vi "Measurement Logic.vi"() -> ()   [LabVIEW 2021, in "Line Regulation_Channel Ganging.lvlib"]
uses:
  Line Regulation_Channel Ganging.lvlib
  Measurement Results.ctl
  <instrlib>/niDCPower/nidcpower.llb/niDCPower Source Mode.ctl
  <instrlib>/niDCPower/nidcpower.llb/niDCPower Output Function.ctl
  <instrlib>/niDCPower/nidcpower.llb/niDCPower Wait For Event - Event.ctl
  shared subVIs/Triggers and Events/NIDCPower_channel_ganging - Configure Digital Edge Source Trigger.vi
  shared subVIs/Triggers and Events/NIDCPower_channel_ganging - Configure Digital Edge Measure Trigger.vi
  <vilib>/Plug-In SDKs/Measurements/Measure Call Context/Measure Call Context.lvclass
  Measurement Configuration.ctl
panel:
  out "measurement results":T1
  in  "measurement configuration":T2={"Source master resource name"="", "Load master resource name"="", "Source slave resource names"=["", ""], "Load slave resource names"=["", ""], "Source system configuration"=enum."Parallel", "Source voltage level range"=64.0, "Source limit symmetry"=enum."Asymmetric", "Source current limit range"=-32.0, "Source current limit low"=-64.0, "Source current limit high"=-64.0, "Source transient response"=1038, "Source sense"=1008, "Source start voltage"=1.0, "Source current sweep points/points per decade"=1, "Source stop voltage"=14.0, "Source voltage gain bandwidth"=2000.0, "Source voltage compensation frequency"=3530.0, "Source voltage pole-zero ratio"=2.0, "Load system configuration"=enum."Parallel", "Load current level"=50.0, "Load current level range"=80.0, "Load limit symmetry"=enum."Symmetric", "Load voltage limit range"=6.0, "Load voltage limit low"=0.0, "Load voltage limit high"=inf, "Load transient response"=1038, "Load sense"=1009, "DUT setup time"=1.0, "Source delay"=0.005, "Aperture time"=0.005, "Load current gain bandwidth"=14000.0, "Load current compensation frequency"=180000.0, "Load current pole-zero ratio"=0.3, "Nominal output voltage"=0.005, "Source sweep type"="Logarithmic"} {"Load sense" items=["Local"=1008, "Remote"=1009]; "Load transient response" items=["Slow"=1041, "Normal"=1038, "Fast"=1039, "Custom"=1042]; "Load voltage limit high" format="%#_6p"; "Load voltage limit low" format="%#_6p"; "Load voltage limit range" format="%#_6p"; "Load current level range" format="%#_6p"; "Source start voltage" format="%#_6p"; "Source sense" items=["Local"=1008, "Remote"=1009]; "Source transient response" items=["Slow"=1041, "Normal"=1038, "Fast"=1039, "Custom"=1042]; "Source current limit low" format="%#_6p"}
  out "measure call context out":refnum<class "Measure Call Context.lvclass">
  in  "measure call context in":refnum<class "Measure Call Context.lvclass">
  out "error out":errorcluster
  in  "error in":errorcluster
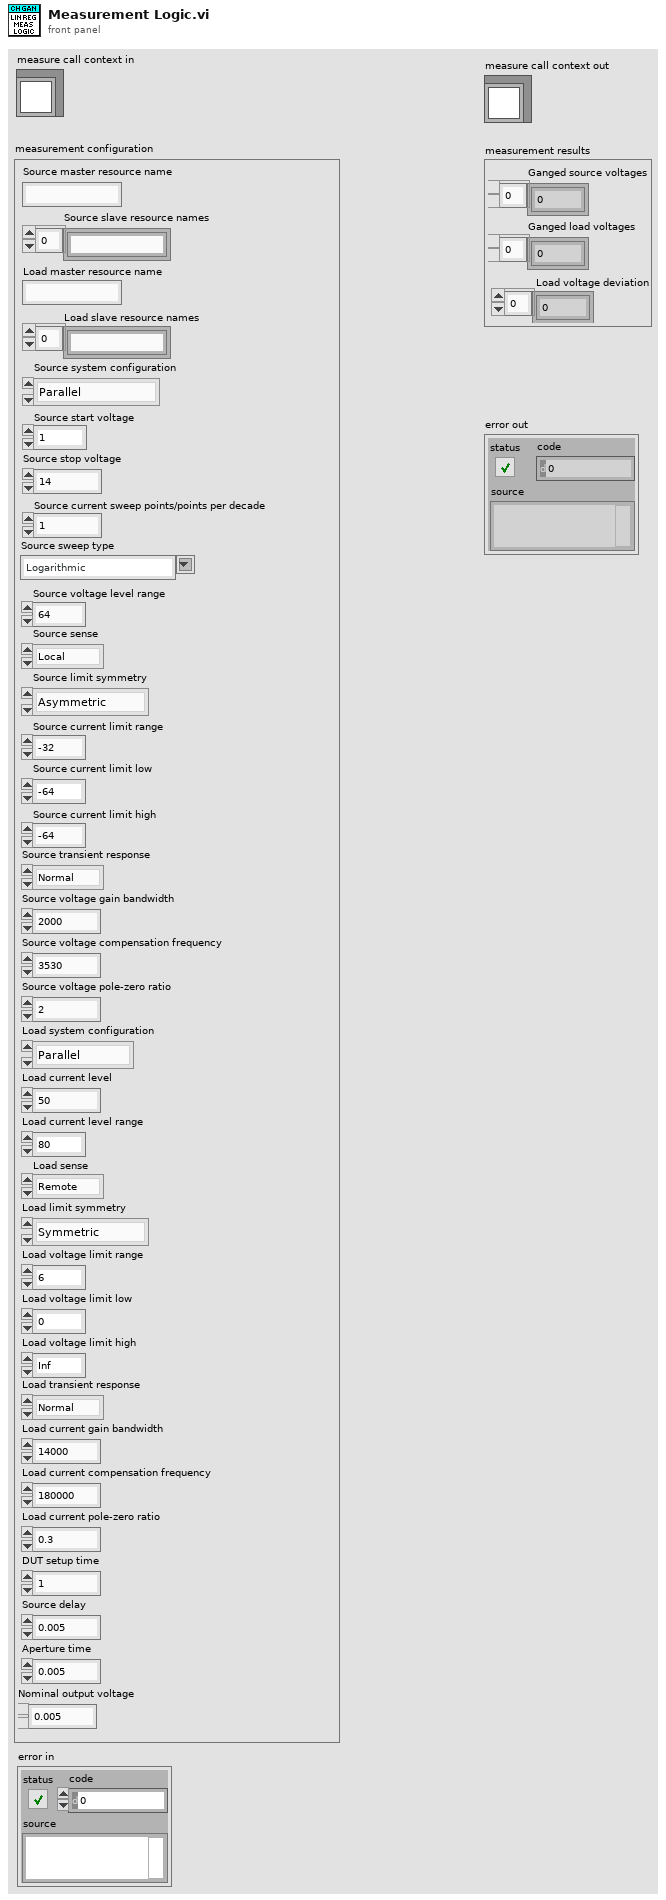
[diagram p1: front panel]
types:
  T1 = typedef "Line Regulation_Channel Ganging.lvlib/Measurement Results.ctl" = cluster{"Ganged source voltages":dbl[], "Ganged load voltages":dbl[], " Load voltage deviation":dbl[]}
  T2 = typedef "Line Regulation_Channel Ganging.lvlib/Measurement Configuration.ctl" = cluster{"Source master resource name":string, "Load master resource name":string, "Source slave resource names":string[], "Load slave resource names":string[], "Source system configuration":enum32{"Series", "Parallel", "Manual"}, "Source voltage level range":dbl, "Source limit symmetry":enum32{"Symmetric", "Asymmetric"}, "Source current limit range":dbl, "Source current limit low":dbl, "Source current limit high":dbl, "Source transient response":i32, "Source sense":i32, "Source start voltage":dbl, "Source current sweep points/points per decade":i32, "Source stop voltage":dbl, "Source voltage gain bandwidth":dbl, "Source voltage compensation frequency":dbl, "Source voltage pole-zero ratio":dbl, "Load system configuration":enum32{"Series", "Parallel", "Manual"}, "Load current level":dbl, "Load current level range":dbl, "Load limit symmetry":enum32{"Symmetric", "Asymmetric"}, "Load voltage limit range":dbl, "Load voltage limit low":dbl, "Load voltage limit high":dbl, "Load transient response":i32, "Load sense":i32, "DUT setup time":dbl, "Source delay":dbl, "Aperture time":dbl, "Load current gain bandwidth":dbl, "Load current compensation frequency":dbl, "Load current pole-zero ratio":dbl, "Nominal output voltage":dbl, "Source sweep type":string}
  T3 = typedef "niDCPower Output Function.ctl" = i32
  T4 = typedef "niDCPower Source Mode.ctl" = i32
  T5 = typedef "niDCPower Wait For Event - Event.ctl" = i32
  T6 = typedef "NIDCPower_channel_ganging - ctl - channel def.ctl" = cluster{"resource name":refnum<k15>, "channels":string, "Channel Mode":T7}
  T7 = typedef "NIDCPower_channel_ganging - ctl - channel mode.ctl" = enum32{"Master", "Slave", "Slave - Inverted"}
  T8 = typedef "NIDCPower_channel_ganging - ctl - ganged session.ctl" = cluster{"Ganged Config":T9, "Session List":refnum<k15>[], "Session Mode":T7[], "Channel":string[]}
  T9 = typedef "NIDCPower_channel_ganging - ctl - ganged config.ctl" = enum32{"Series", "Parallel", "Manual"}
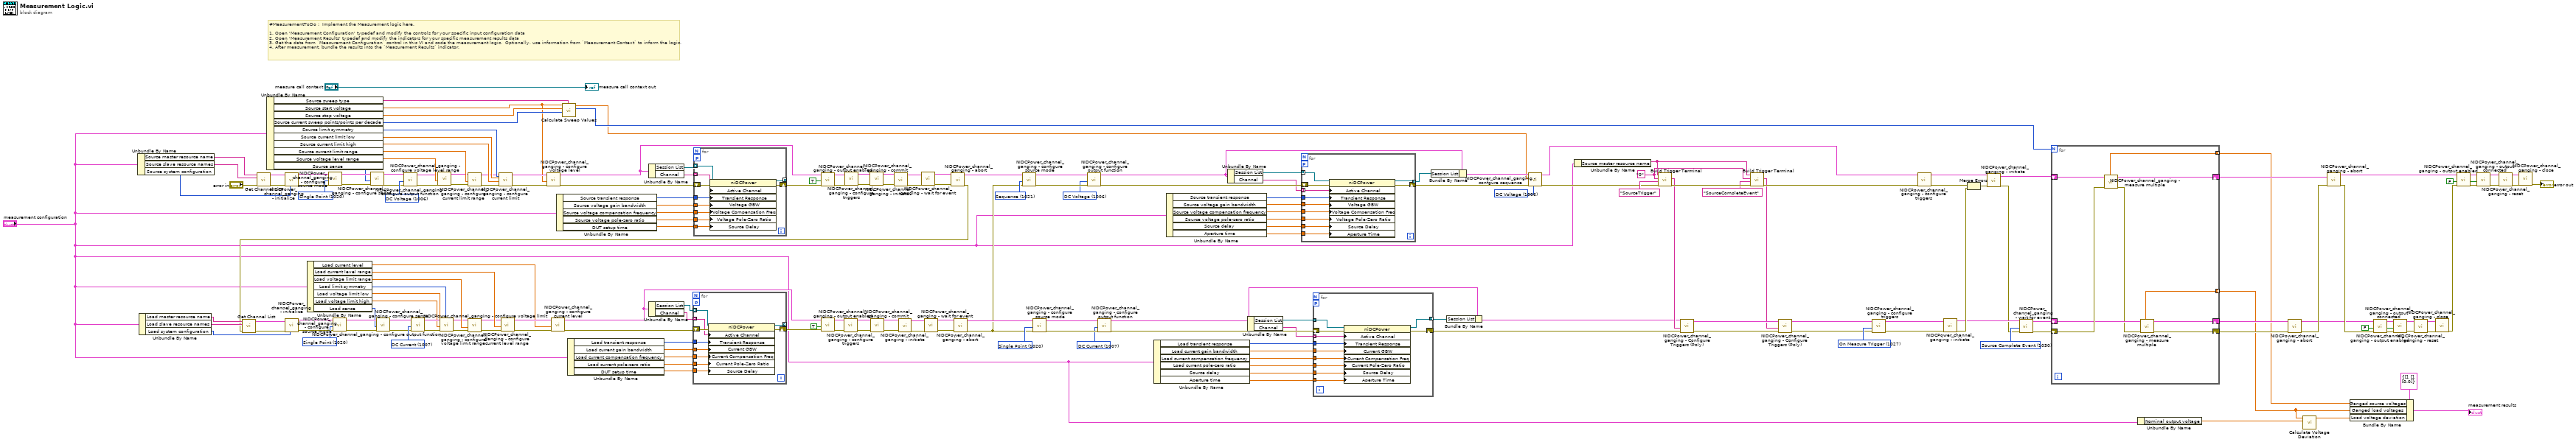
[diagram p0: block diagram]
diagram:
  w37 = T3 1006 items=["DC Voltage"=1006, "DC Current"=1007, "Pulse Voltage"=1049, "Pulse Current"=1050] ("output function")
  w60 = "0" ("Channel Name")
  w95 = 1027 items=["Automatically after Source Complete"=1025, "On Demand"=1026, "On Measure Trigger"=1027] ("Measure When")
  w92 = T3 1006 items=["DC Voltage"=1006, "DC Current"=1007, "Pulse Voltage"=1049, "Pulse Current"=1050] ("output function")
  w97 = T4 1021 items=["Single Point"=1020, "Sequence"=1021] ("source mode")
  w98 = T4 1020 items=["Single Point"=1020, "Sequence"=1021] ("source mode")
  w44 = T3 1007 items=["DC Voltage"=1006, "DC Current"=1007, "Pulse Voltage"=1049, "Pulse Current"=1050] ("output function")
  w145 = T5 1030 items=["Source Complete Event"=1030, "Measure Complete Event"=1031, "Sequence Iteration Complete Event"=1032, "Sequence Engine Done Event"=1033, "Pulse Complete Event"=1051, "Ready For Pulse Trigger Event"=1052] ("event")
  w146 = T3 1007 items=["DC Voltage"=1006, "DC Current"=1007, "Pulse Voltage"=1049, "Pulse Current"=1050] ("output function")
  w159 = T3 1006 items=["DC Voltage"=1006, "DC Current"=1007, "Pulse Voltage"=1049, "Pulse Current"=1050] ("output function")
  w165 = FALSE ("output enabled")
  w164 = FALSE ("output enabled")
  w197 = T4 1020 items=["Single Point"=1020, "Sequence"=1021] ("source mode")
  w198 = T4 1020 items=["Single Point"=1020, "Sequence"=1021] ("source mode")
  # "#MeasurementToDo :  Implement the Measurement logic here.\n\n1. Open 'Measurement Configuration' typedef and modify the controls for your specific input configuration data\n2. Open 'Measurement Results' typedef and modify the indicators for your specific measurement results data\n3. Get the data from `Measurement Configuration` control in this VI and code the measurement logic.  Optionally, use information from `Measurement Context` to inform the logic.\n4. After measurement, bundle the results into the `Measurement Results` indicator."
  n1 = Unbundle By Name("measurement configuration") -> ("Source master resource name"=w53:string, "Source slave resource names"=w52:string[], "Source system configuration"=w176:enum32{"Series", "Parallel", "Manual"})
  n2 = Unbundle By Name("measurement configuration") -> ("Load master resource name"=w49:string, "Load slave resource names"=w48:string[], "Load system configuration"=w175:enum32{"Series", "Parallel", "Manual"})
  n3 = call "Get Channel List.vi"("error in (no error)"="error in", "Slave resource names"=w52, "Master resouce name"=w53) -> ("error out"=w54:errorcluster, "Channel List"=w55:T6[])  [unwired: 7 in]
  n4 = Unbundle By Name("measurement configuration") -> ("Source sweep type"=w6:string, "Source start voltage"=w7:dbl, "Source stop voltage"=w11:dbl, "Source current sweep points/points per decade"=w10:i32, "Source limit symmetry"=w182:enum32{"Symmetric", "Asymmetric"}, "Source current limit low"=w183:dbl, "Source current limit high"=w184:dbl, "Source current limit range"=w185:dbl, "Source voltage level range"=w186:dbl, "Source sense"=w58:i32)
  n5 = call "NIDCPower_channel_ganging - initialize.vi"("Ganged Config"=w176, "error in (no error)"=w54, "Channel List"=w55) -> ("error out"=w199:errorcluster, "Ganged Session Out"=w200:T8)  [unwired: 7 in]
  n6 = Unbundle By Name("measurement configuration") -> ("Load current level"=w65:dbl, "Load current level range"=w177:dbl, "Load voltage limit range"=w178:dbl, "Load limit symmetry"=w181:enum32{"Symmetric", "Asymmetric"}, "Load voltage limit low"=w180:dbl, "Load voltage limit high"=w179:dbl, "Load sense"=w59:i32)
  n7 = call "NIDCPower_channel_ganging - configure source mode.vi"("error in (no error)"=w199, "source mode"=w198, "Ganged Session In"=w200) -> ("error out"=w142:errorcluster, "Ganged Session Out"=w143:T8)  [unwired: 7 in]
  n8 = call "NIDCPower_channel_ganging - configure sense.vi"("error in (no error)"=w142, "sense"=w58, "Ganged Session In"=w143) -> ("error out"=w140:errorcluster, "Ganged Session Out"=w141:T8)  [unwired: 7 in]
  n9 = call "NIDCPower_channel_ganging - configure output function.vi"("error in (no error)"=w140, "output function"=w159, "Ganged Session In"=w141) -> ("error out"=w138:errorcluster, "Ganged Session Out"=w139:T8)  [unwired: 7 in]
  n10 = call "NIDCPower_channel_ganging - configure voltage level range.vi"("error in (no error)"=w138, "voltage level range"=w186, "Ganged Session In"=w139) -> ("error out"=w155:errorcluster, "Ganged Session Out"=w158:T8)  [unwired: 7 in]
  n11 = call "NIDCPower_channel_ganging - configure current limit range.vi"("error in (no error)"=w155, "current limit range"=w185, "Ganged Session In"=w158) -> ("error out"=w154:errorcluster, "Ganged Session Out"=w157:T8)  [unwired: 7 in]
  n12 = call "NIDCPower_channel_ganging - configure current limit.vi"("Limit Symmetry"=w182, "error in (no error)"=w154, "Current limit/hi"=w184, "Current limit lo"=w183, "Ganged Session In"=w157) -> ("error out"=w153:errorcluster, "Ganged Session Out"=w156:T8)  [unwired: 5 in]
  n13 = call "NIDCPower_channel_ganging - configure voltage level.vi"("error in (no error)"=w153, "voltage level"=w7, "Ganged Session In"=w156) -> ("error out"=w113:errorcluster, "Ganged Session Out"=w107:T8)  [unwired: 7 in]
  n14 = Unbundle By Name("measurement configuration") -> ("Source transient response"=w31:i32, "Source voltage gain bandwidth"=w27:dbl, "Source voltage compensation frequency"=w26:dbl, "Source voltage pole-zero ratio"=w25:dbl, "DUT setup time"=w28:dbl)
  n15 = call "Calculate Sweep Values.vi"("Sweep type"=w6, "Points"=w10, "Stop level"=w11, "Start level"=w7) -> ("Sweep points"=w9:i32, "Sweep values"=w8:dbl[])  [unwired: 5 in, 1 out]
  n16 = Unbundle By Name("measurement configuration") -> ("Load transient response"=w30:i32, "Load current gain bandwidth"=w24:dbl, "Load current compensation frequency"=w23:dbl, "Load current pole-zero ratio"=w22:dbl, "DUT setup time"=w29:dbl)
  n17 = Unbundle By Name(w107) -> ("Session List"=w111:refnum<k15>[], "Channel"=w110:string[])
  n18 = for {
    tunnel: [w211] -> _ mode=indexing
    shift-right: [w209] -> w112
    shift-left: w113 -> [w210]
    workers-P: _ -> [_]
    tunnel: w111 -> [w208] mode=indexing
    tunnel: w110 -> [w207] mode=indexing
    tunnel: w31 -> [w206]
    tunnel: w28 -> [w205]
    tunnel: w27 -> [w204]
    tunnel: w26 -> [w203]
    tunnel: w25 -> [w202]
    n19 = property class="niDCPower"(reference=w208, error in=w210, "Active Channel"=w207, "Transient Response"=w206, "Voltage GBW"=w204, "Voltage Compensation Freq"=w203, "Voltage Pole-Zero Ratio"=w202, "Source Delay"=w205) -> (reference out=w211:refnum<k15>, error out=w209:errorcluster)
  }
  n20 = call "NIDCPower_channel_ganging - output enabled.vi"("error in (no error)"=w112, "output enabled"=TRUE, "Ganged Session In"=w107) -> ("error out"=w116:errorcluster, "Ganged Session Out"=w117:T8)  [unwired: 7 in]
  n21 = call "NIDCPower_channel_ganging - configure triggers.vi"("error in (no error)"=w116, "Ganged Session In"=w117) -> ("error out"=w114:errorcluster, "Ganged Session Out"=w115:T8)  [unwired: 8 in]
  n22 = call "NIDCPower_channel_ganging - commit.vi"("error in (no error)"=w114, "Ganged Session In"=w115) -> ("error out"=w123:errorcluster, "Ganged Session Out"=w122:T8)  [unwired: 8 in]
  n23 = call "NIDCPower_channel_ganging - initiate.vi"("error in (no error)"=w123, "Ganged Session In"=w122) -> ("error out"=w125:errorcluster, "Ganged Session Out"=w124:T8)  [unwired: 8 in]
  n24 = call "NIDCPower_channel_ganging - wait for event.vi"("error in (no error)"=w125, "Ganged Session in"=w124) -> ("error out"=w127:errorcluster, "Ganged Session Out"=w126:T8)  [unwired: 8 in]
  n25 = call "NIDCPower_channel_ganging - abort.vi"("error in (no error)"=w127, "Ganged Session In"=w126) -> ("error out"=w47:errorcluster, "Ganged Session Out"=w96:T8)  [unwired: 8 in]
  n26 = call "Get Channel List.vi"("error in (no error)"=w47, "Slave resource names"=w48, "Master resouce name"=w49) -> ("error out"=w51:errorcluster, "Channel List"=w50:T6[])  [unwired: 7 in]
  n27 = call "NIDCPower_channel_ganging - initialize.vi"("Ganged Config"=w175, "error in (no error)"=w51, "Channel List"=w50) -> ("error out"=w196:errorcluster, "Ganged Session Out"=w195:T8)  [unwired: 7 in]
  n28 = call "NIDCPower_channel_ganging - configure source mode.vi"("error in (no error)"=w196, "source mode"=w197, "Ganged Session In"=w195) -> ("error out"=w136:errorcluster, "Ganged Session Out"=w137:T8)  [unwired: 7 in]
  n29 = call "NIDCPower_channel_ganging - configure sense.vi"("error in (no error)"=w136, "sense"=w59, "Ganged Session In"=w137) -> ("error out"=w134:errorcluster, "Ganged Session Out"=w135:T8)  [unwired: 7 in]
  n30 = call "NIDCPower_channel_ganging - configure output function.vi"("error in (no error)"=w134, "output function"=w146, "Ganged Session In"=w135) -> ("error out"=w193:errorcluster, "Ganged Session Out"=w194:T8)  [unwired: 7 in]
  n31 = call "NIDCPower_channel_ganging - configure voltage limit.vi"("Limit Symmetry"=w181, "error in (no error)"=w193, "voltage limit/hi"=w179, "voltage limit lo"=w180, "Ganged Session In"=w194) -> ("error out"=w151:errorcluster, "Ganged Session Out"=w152:T8)  [unwired: 5 in]
  n32 = call "NIDCPower_channel_ganging - configure voltage limit range.vi"("error in (no error)"=w151, "voltage level range"=w178, "Ganged Session In"=w152) -> ("error out"=w149:errorcluster, "Ganged Session Out"=w150:T8)  [unwired: 7 in]
  n33 = call "NIDCPower_channel_ganging - configure current level range.vi"("error in (no error)"=w149, "current level range"=w177, "Ganged Session In"=w150) -> ("error out"=w147:errorcluster, "Ganged Session Out"=w148:T8)  [unwired: 7 in]
  n34 = call "NIDCPower_channel_ganging - configure current level.vi"("error in (no error)"=w147, "current level"=w65, "Ganged Session In"=w148) -> ("error out"=w109:errorcluster, "Ganged Session Out"=w106:T8)  [unwired: 7 in]
  n35 = Unbundle By Name(w106) -> ("Session List"=w105:refnum<k15>[], "Channel"=w104:string[])
  n36 = for {
    tunnel: [w221] -> _ mode=indexing
    shift-right: [w219] -> w108
    shift-left: w109 -> [w220]
    workers-P: _ -> [_]
    tunnel: w105 -> [w218] mode=indexing
    tunnel: w104 -> [w217] mode=indexing
    tunnel: w30 -> [w216]
    tunnel: w29 -> [w215]
    tunnel: w24 -> [w214]
    tunnel: w23 -> [w213]
    tunnel: w22 -> [w212]
    n37 = property class="niDCPower"(reference=w218, error in=w220, "Active Channel"=w217, "Transient Response"=w216, "Current GBW"=w214, "Current Compensation Freq"=w213, "Current Pole-Zero Ratio"=w212, "Source Delay"=w215) -> (reference out=w221:refnum<k15>, error out=w219:errorcluster)
  }
  n38 = call "NIDCPower_channel_ganging - output enabled.vi"("error in (no error)"=w108, "output enabled"=TRUE, "Ganged Session In"=w106) -> ("error out"=w120:errorcluster, "Ganged Session Out"=w121:T8)  [unwired: 7 in]
  n39 = call "NIDCPower_channel_ganging - configure triggers.vi"("error in (no error)"=w120, "Ganged Session In"=w121) -> ("error out"=w118:errorcluster, "Ganged Session Out"=w119:T8)  [unwired: 8 in]
  n40 = call "NIDCPower_channel_ganging - commit.vi"("error in (no error)"=w118, "Ganged Session In"=w119) -> ("error out"=w132:errorcluster, "Ganged Session Out"=w133:T8)  [unwired: 8 in]
  n41 = call "NIDCPower_channel_ganging - initiate.vi"("error in (no error)"=w132, "Ganged Session In"=w133) -> ("error out"=w130:errorcluster, "Ganged Session Out"=w131:T8)  [unwired: 8 in]
  n42 = call "NIDCPower_channel_ganging - wait for event.vi"("error in (no error)"=w130, "Ganged Session in"=w131) -> ("error out"=w128:errorcluster, "Ganged Session Out"=w129:T8)  [unwired: 8 in]
  n43 = call "NIDCPower_channel_ganging - abort.vi"("error in (no error)"=w128, "Ganged Session In"=w129) -> ("error out"=w70:errorcluster, "Ganged Session Out"=w99:T8)  [unwired: 8 in]
  n44 = call "NIDCPower_channel_ganging - configure source mode.vi"("error in (no error)"=w70, "source mode"=w97, "Ganged Session In"=w96) -> ("error out"=w100:errorcluster, "Ganged Session Out"=w101:T8)  [unwired: 7 in]
  n45 = call "NIDCPower_channel_ganging - configure source mode.vi"("error in (no error)"=w70, "source mode"=w98, "Ganged Session In"=w99) -> ("error out"=w103:errorcluster, "Ganged Session Out"=w102:T8)  [unwired: 7 in]
  n46 = call "NIDCPower_channel_ganging - configure output function.vi"("error in (no error)"=w100, "output function"=w92, "Ganged Session In"=w101) -> ("error out"=w93:errorcluster, "Ganged Session Out"=w94:T8)  [unwired: 7 in]
  n47 = call "NIDCPower_channel_ganging - configure output function.vi"("error in (no error)"=w103, "output function"=w44, "Ganged Session In"=w102) -> ("error out"=w75:errorcluster, "Ganged Session Out"=w76:T8)  [unwired: 7 in]
  n48 = Unbundle By Name("measurement configuration") -> ("Load transient response"=w36:i32, "Load current gain bandwidth"=w18:dbl, "Load current compensation frequency"=w17:dbl, "Load current pole-zero ratio"=w16:dbl, "Source delay"=w35:dbl, "Aperture time"=w34:dbl)
  n49 = Unbundle By Name("measurement configuration") -> ("Source transient response"=w38:i32, "Source voltage gain bandwidth"=w21:dbl, "Source voltage compensation frequency"=w20:dbl, "Source voltage pole-zero ratio"=w19:dbl, "Source delay"=w33:dbl, "Aperture time"=w32:dbl)
  n50 = Unbundle By Name(w94) -> ("Session List"=w190:refnum<k15>[], "Channel"=w74:string[])
  n51 = Unbundle By Name(w76) -> ("Session List"=w73:refnum<k15>[], "Channel"=w72:string[])
  n52 = for {
    tunnel: [w232] -> w189 mode=indexing
    shift-right: [w230] -> w41
    shift-left: w93 -> [w231]
    workers-P: _ -> [_]
    tunnel: w190 -> [w229] mode=indexing
    tunnel: w74 -> [w228] mode=indexing
    tunnel: w38 -> [w227]
    tunnel: w33 -> [w226]
    tunnel: w32 -> [w225]
    tunnel: w21 -> [w224]
    tunnel: w20 -> [w223]
    tunnel: w19 -> [w222]
    n53 = property class="niDCPower"(reference=w229, error in=w231, "Active Channel"=w228, "Transient Response"=w227, "Voltage GBW"=w224, "Voltage Compensation Freq"=w223, "Voltage Pole-Zero Ratio"=w222, "Source Delay"=w226, "Aperture Time"=w225) -> (reference out=w232:refnum<k15>, error out=w230:errorcluster)
  }
  n54 = for {
    tunnel: [w243] -> w71 mode=indexing
    shift-right: [w241] -> w45
    shift-left: w75 -> [w242]
    workers-P: _ -> [_]
    tunnel: w73 -> [w240] mode=indexing
    tunnel: w72 -> [w239] mode=indexing
    tunnel: w36 -> [w238]
    tunnel: w35 -> [w237]
    tunnel: w34 -> [w236]
    tunnel: w18 -> [w235]
    tunnel: w17 -> [w234]
    tunnel: w16 -> [w233]
    n55 = property class="niDCPower"(reference=w240, error in=w242, "Active Channel"=w239, "Transient Response"=w238, "Current GBW"=w235, "Current Compensation Freq"=w234, "Current Pole-Zero Ratio"=w233, "Source Delay"=w237, "Aperture Time"=w236) -> (reference out=w243:refnum<k15>, error out=w241:errorcluster)
  }
  n56 = Bundle By Name(cluster=w94, "Session List"=w189) -> (w43:T8)
  n57 = Bundle By Name(cluster=w76, "Session List"=w71) -> (w46:T8)
  n58 = call "NIDCPower_channel_ganging - confgure sequence.vi"("output function"=w37, "error in (no error)"=w41, "Values"=w8, "Ganged Session In"=w43) -> ("error out"=w40:errorcluster, "Ganged Session Out"=w42:T8)  [unwired: 6 in]
  n59 = Unbundle By Name("measurement configuration") -> ("Source master resource name"=w39:string)
  n60 = call "Build Trigger Terminal.vi"("error in (no error)"=w40, "Trigger/Event Name"="SourceTrigger", "Channel Name"=w60, "Resource Name"=w39) -> ("error out"=w69:errorcluster, "Terminal Name"=w57:string)  [unwired: 6 in]
  n61 = call-poly "NIDCPower_channel_ganging - Configure Triggers (Poly).vi"("error in (no error)"=w45, "output terminal"=w57, "Ganged Session in"=w46) -> ("error out"=w61:errorcluster, "Ganged Session out"=w62:T8)  [unwired: 7 in]
  n62 = call "Build Trigger Terminal.vi"("error in (no error)"=w69, "Trigger/Event Name"="SourceCompleteEvent", "Channel Name"=w60, "Resource Name"=w39) -> ("error out"=w68:errorcluster, "Terminal Name"=w56:string)  [unwired: 6 in]
  n63 = call-poly "NIDCPower_channel_ganging - Configure Triggers (Poly).vi"("error in (no error)"=w61, "output terminal"=w56, "Ganged Session in"=w62) -> ("error out"=w63:errorcluster, "Ganged Session out"=w64:T8)  [unwired: 7 in]
  n64 = call "NIDCPower_channel_ganging - configure triggers.vi"("error in (no error)"=w63, "Measure When"=w95, "Ganged Session In"=w64) -> ("error out"=w187:errorcluster, "Ganged Session Out"=w188:T8)  [unwired: 7 in]
  n65 = call "NIDCPower_channel_ganging - configure triggers.vi"("error in (no error)"=w68, "Ganged Session In"=w42) -> ("error out"=w161:errorcluster, "Ganged Session Out"=w162:T8)  [unwired: 8 in]
  n66 = call "NIDCPower_channel_ganging - initiate.vi"("error in (no error)"=w187, "Ganged Session In"=w188) -> ("error out"=w160:errorcluster, "Ganged Session Out"=w144:T8)  [unwired: 8 in]
  n67 = Merge Errors(w161, w160) -> (w163:errorcluster)
  n68 = call "NIDCPower_channel_ganging - initiate.vi"("error in (no error)"=w163, "Ganged Session In"=w162) -> ("error out"=w91:errorcluster, "Ganged Session Out"=w78:T8)  [unwired: 8 in]
  n69 = call "NIDCPower_channel_ganging - wait for event.vi"("error in (no error)"=w91, "event"=w145, "Ganged Session in"=w144) -> ("error out"=w82:errorcluster, "Ganged Session Out"=w80:T8)  [unwired: 7 in]
  n70 = for {
    N: w9 -> [_]
    shift-right: [w251] -> w81
    shift-left: w82 -> [w252]
    shift-right: [w249] -> w79
    shift-left: w80 -> [w250]
    shift-right: [w247] -> w77
    shift-left: w78 -> [w248]
    tunnel: [w245] -> w13 mode=indexing
    tunnel: [w244] -> w4 mode=indexing
    n71 = call "NIDCPower_channel_ganging - measure multiple.vi"("error in (no error)"=w252, "Ganged Session In"=w248) -> ("error out"=w246:errorcluster, "Ganged Session Out"=w247:T8, "ganged voltage measurement"=w245:dbl)  [unwired: 2 in, 5 out]
    n72 = call "NIDCPower_channel_ganging - measure multiple.vi"("error in (no error)"=w246, "Ganged Session In"=w250) -> ("error out"=w251:errorcluster, "Ganged Session Out"=w249:T8, "ganged voltage measurement"=w244:dbl)  [unwired: 2 in, 5 out]
  }
  n73 = Unbundle By Name("measurement configuration") -> ("Nominal output voltage"=w5:dbl)
  n74 = call "NIDCPower_channel_ganging - abort.vi"("error in (no error)"=w81, "Ganged Session In"=w79) -> ("error out"=w174:errorcluster, "Ganged Session Out"=w170:T8)  [unwired: 8 in]
  n75 = call "Calculate Voltage Deviation.vi"("Nominal output voltage"=w5, "Voltage measurements"=w4) -> ("Load voltage deviation"=w3:dbl[])  [unwired: 9 in]
  n76 = call "NIDCPower_channel_ganging - abort.vi"("error in (no error)"=w174, "Ganged Session In"=w77) -> ("error out"=w173:errorcluster, "Ganged Session Out"=w166:T8)  [unwired: 8 in]
  n77 = Bundle By Name(cluster=T1 {"Ganged source voltages"=[], "Ganged load voltages"=[], " Load voltage deviation"=[0.0]} ("Measurement Results"), "Ganged source voltages"=w13, "Ganged load voltages"=w4, "Load voltage deviation"=w3) -> (→"measurement results":T1)
  n78 = call "NIDCPower_channel_ganging - output enabled.vi"("error in (no error)"=w173, "output enabled"=w165, "Ganged Session In"=w170) -> ("error out"=w171:errorcluster, "Ganged Session Out"=w172:T8)  [unwired: 7 in]
  n79 = call "NIDCPower_channel_ganging - output connected.vi"("error in (no error)"=w171, "output enabled"=w165, "Ganged Session In"=w172) -> ("error out"=w90:errorcluster, "Ganged Session Out"=w89:T8)  [unwired: 7 in]
  n80 = call "NIDCPower_channel_ganging - reset.vi"("error in (no error)"=w90, "Ganged Session In"=w89) -> ("error out"=w87:errorcluster, "Ganged Session Out"=w88:T8)  [unwired: 8 in]
  n81 = call "NIDCPower_channel_ganging - close.vi"("error in (no error)"=w87, "Ganged Session In"=w88) -> ("error out"=w167:errorcluster)  [unwired: 9 in]
  n82 = call "NIDCPower_channel_ganging - output enabled.vi"("error in (no error)"=w167, "output enabled"=w164, "Ganged Session In"=w166) -> ("error out"=w169:errorcluster, "Ganged Session Out"=w168:T8)  [unwired: 7 in]
  n83 = call "NIDCPower_channel_ganging - output connected.vi"("error in (no error)"=w169, "output enabled"=w164, "Ganged Session In"=w168) -> ("error out"=w85:errorcluster, "Ganged Session Out"=w86:T8)  [unwired: 7 in]
  n84 = call "NIDCPower_channel_ganging - reset.vi"("error in (no error)"=w85, "Ganged Session In"=w86) -> ("error out"=w83:errorcluster, "Ganged Session Out"=w84:T8)  [unwired: 8 in]
  n85 = call "NIDCPower_channel_ganging - close.vi"("error in (no error)"=w83, "Ganged Session In"=w84) -> ("error out"=→"error out":errorcluster)  [unwired: 9 in]
  "measure call context out" <- "measure call context in"
